vi "Aumento Credito.vi"(8 "error in (no error)":errorcluster, 10 "Dinero":i32, 11 "Dinero in":refnum<class "Dinero.lvclass">) -> (0 "error out":errorcluster, 3 "Dinero out":refnum<class "Dinero.lvclass">)   [LabVIEW 2020, in "Dinero.lvlib" / "Dinero.lvclass"]
uses:
  Dinero.lvclass
  C:/Program Files (x86)/National Instruments/LabVIEW 2020/vi.lib/ActorFramework/Actor/Actor.lvclass
  Dinero.lvclass/Dinero.ctl
  <vilib>/ActorFramework/Actor/Actor.lvclass/Actor.ctl
  UI Messages/Obtain Credito from Dinero Msg/Obtain Credito from Dinero Msg.lvclass/Obtain Credito from Dinero Msg.ctl
  <vilib>/ActorFramework/Message Enqueuer/Message Enqueuer.lvclass/Message Enqueuer.ctl
  <vilib>/ActorFramework/Message Enqueuer/Enqueue.vi
  UI Messages/Obtain Credito from Dinero Msg/Obtain Credito from Dinero Msg.lvclass
  C:/Program Files (x86)/National Instruments/LabVIEW 2020/vi.lib/ActorFramework/Message/Message.lvclass
  <vilib>/ActorFramework/Message Priority Queue/Priority Enqueue.vi
  <vilib>/ActorFramework/Actor/Actor.lvclass
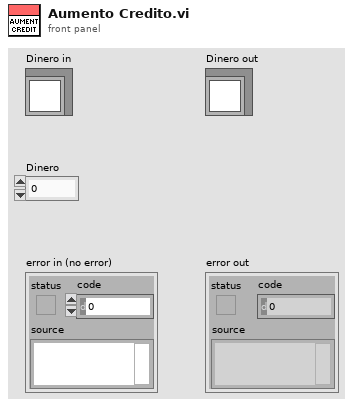
[diagram p1: front panel]
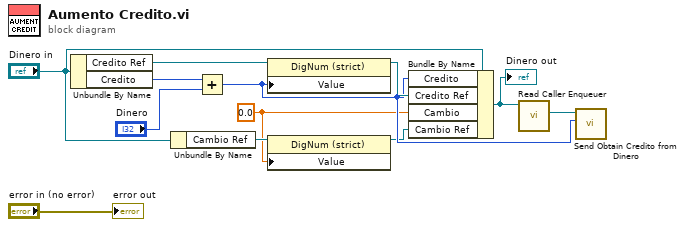
[diagram p0: block diagram]
diagram:
  w1 = 0.0 ("Value")
  n1 = Unbundle By Name("Dinero in") -> ("Credito Ref"=w11:refnum<vi>, "Credito"=w9:i32)
  n2 = Unbundle By Name("Dinero in") -> ("Cambio Ref"=w3:refnum<vi>)
  n3 = Add(x=w9, y="Dinero") -> (x+y=w5:i32)
  n4 = property class="DigNum (strict)"(reference=w11, "Value"=w5) -> (reference out=w10:refnum<vi>)  [unwired: 1 in, 1 out]
  n5 = property class="DigNum (strict)"(reference=w3, "Value"=w1) -> (reference out=w2:refnum<vi>)  [unwired: 1 in, 1 out]
  n6 = Bundle By Name(cluster="Dinero in", "Credito"=w5, "Credito Ref"=w10, "Cambio"=w1, "Cambio Ref"=w2) -> (w7:refnum<class "Dinero.lvclass">)
  "Dinero out" <- w7
  n7 = call <vilib>:"Read Caller Enqueuer.vi"("Actor"=w7) -> ("Caller Enqueuer"=w6:refnum<class "Message Enqueuer.lvclass">)  [unwired: 10 in]
  n8 = call "Send Obtain Credito from Dinero.vi"("Credito"=w5, "Message Enqueuer"=w6) -> ()  [unwired: 8 in, 2 out]
  "error out" <- "error in (no error)"
